vi "SVPWMTimingabcSGL01_src.vi"(0 "A":sgl, 1 "tm":sgl, 2 "tmDIVvdc":sgl, 5 "B":sgl, 7 "C":sgl) -> (4 "U":sgl, 6 "V":sgl, 8 "W":sgl, 14 "Sector":u8)   [LabVIEW 2015]
panel:
  out "tz":sgl
  out "ty":sgl
  out "tx":sgl
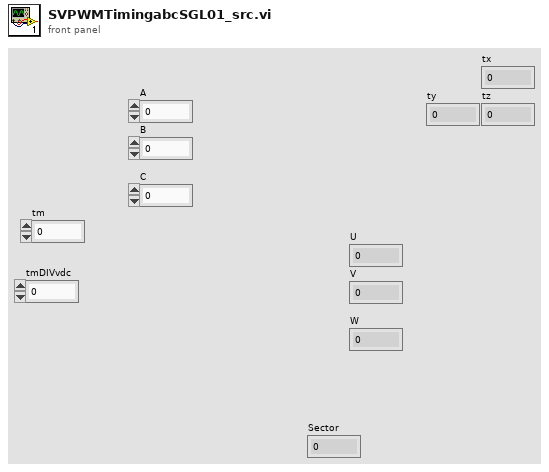
[diagram p1: front panel]
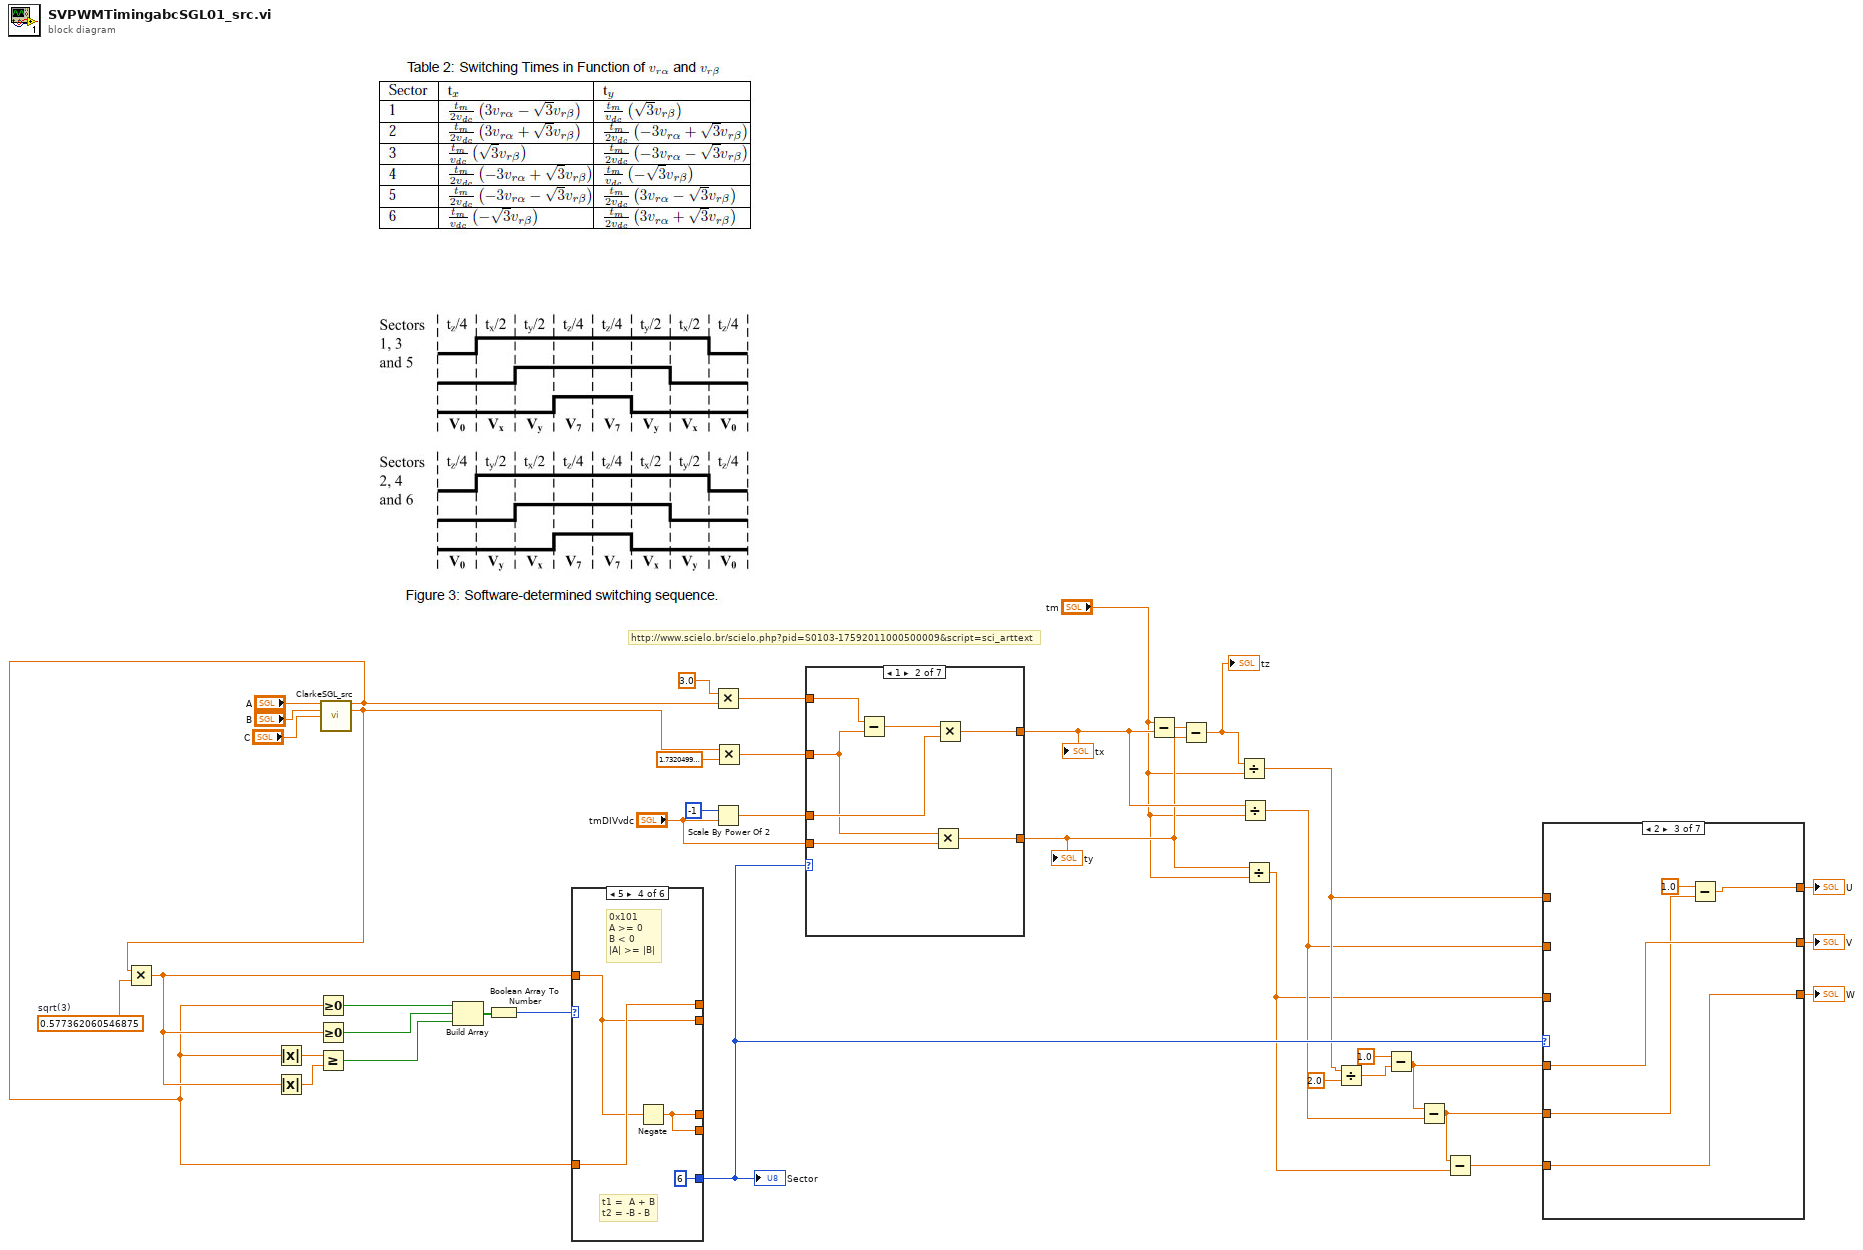
[diagram p0: block diagram]
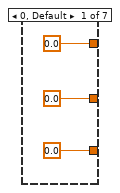
[diagram p2: hidden frame]
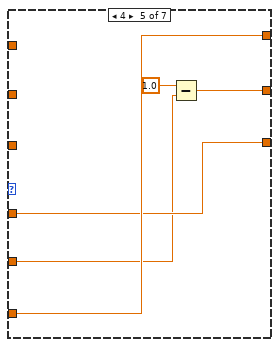
[diagram p5: hidden frame]
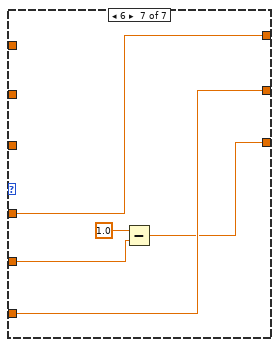
[diagram p7: hidden frame]
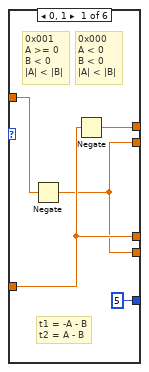
[diagram p8: hidden frame]
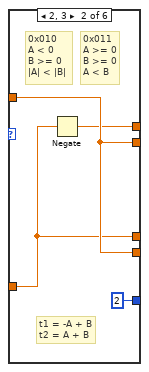
[diagram p9: hidden frame]
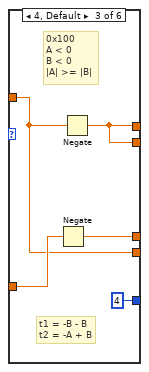
[diagram p10: hidden frame]
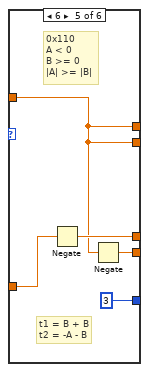
[diagram p11: hidden frame]
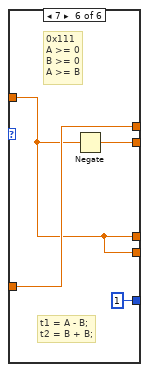
[diagram p12: hidden frame]
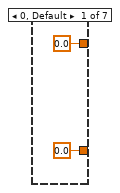
[diagram p13: hidden frame]
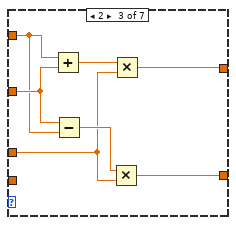
[diagram p14: hidden frame]
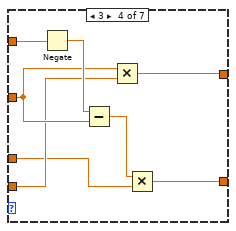
[diagram p15: hidden frame]
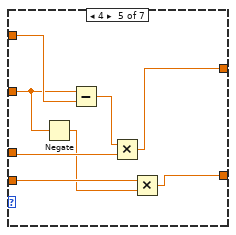
[diagram p16: hidden frame]
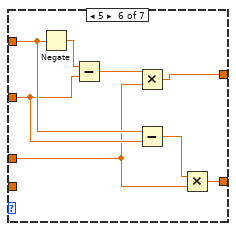
[diagram p17: hidden frame]
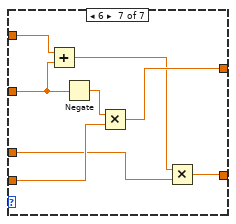
[diagram p18: hidden frame]
diagram:
  w27 = sgl 0.57736206  # sqrt(3)
  # "http://www.scielo.br/scielo.php?pid=S0103-17592011000500009&script=sci_arttext"
  n1 = call "ClarkeSGL_src.vi"("A"="A", "B"="B", "C"="C") -> ("alpha"=w19:sgl, "beta"=w20:sgl)  [unwired: 11 in]
  n2 = Multiply(x=w20, y=w27) -> (x*y=w28:sgl)
  n3 = Absolute Value(x=w19) -> (abs(x)=w26:sgl)
  n4 = Absolute Value(x=w28) -> (abs(x)=w25:sgl)
  n5 = Greater Or Equal To 0?(x=w19) -> (x >= 0?=w23:bool)
  n6 = Greater Or Equal To 0?(x=w28) -> (x >= 0?=w22:bool)
  n7 = Greater Or Equal?(x=w26, y=w25) -> (x >= y?=w21:bool)
  n8 = Build Array(w23, w22, w21) -> (w24:bool[])
  n9 = Boolean Array To Number(Boolean array=w24) -> (number=w29:u8)
  n10 = case shown="5" w29 {
    tunnel: w28 -> [w44 w48 w50 w56 w60 w64]
    tunnel: w19 -> [w42 w46 w53 w57 w62 w65]
    tunnel: [w43 w47 w51 w57 w60 w65] -> _
    tunnel: [w41 w48 w51 w56 w60 w66] -> _
    tunnel: [w42 w46 w52 w55 w61 w64] -> _
    tunnel: [w41 w48 w50 w55 w59 w64] -> _
    tunnel: [u8 5 u8 2 u8 4 u8 6 u8 3 u8 1] -> w17
    frame 0, 1 {
      # "0x000\nA < 0\nB < 0\n|A| < |B|"
      # "t1 = -A - B\nt2 = A - B"
      # "0x001\nA >= 0\nB < 0\n|A| < |B|"
      n11 = Negate(x=w44) -> (-x=w41:sgl)
      n12 = Negate(x=w42) -> (-x=w43:sgl)
    }
    frame 2, 3 {
      # "0x011\nA >= 0\nB >= 0\nA < B"
      # "t1 = -A + B\nt2 = A + B"
      # "0x010\nA < 0\nB >= 0\n|A| < |B|"
      n13 = Negate(x=w46) -> (-x=w47:sgl)
    }
    frame 4, Default {
      # "t1 = -B - B\nt2 = -A + B"
      # "0x100\nA < 0\nB < 0\n|A| >= |B|"
      n14 = Negate(x=w53) -> (-x=w52:sgl)
      n15 = Negate(x=w50) -> (-x=w51:sgl)
    }
    frame 5 {
      # "t1 =  A + B\nt2 = -B - B"
      # "0x101\nA >= 0\nB < 0\n|A| >= |B|"
      n16 = Negate(x=w56) -> (-x=w55:sgl)
    }
    frame 6 {
      # "t1 = B + B\nt2 = -A - B"
      # "0x110\nA < 0\nB >= 0\n|A| >= |B|"
      n17 = Negate(x=w62) -> (-x=w61:sgl)
      n18 = Negate(x=w60) -> (-x=w59:sgl)
    }
    frame 7 {
      # "t1 = A - B;\nt2 = B + B;"
      # "0x111\nA >= 0\nB >= 0\nA >= B"
      n19 = Negate(x=w64) -> (-x=w66:sgl)
    }
  }
  "Sector" <- w17
  n20 = Multiply(x=sgl 3.0, y=w19) -> (x*y=w33:sgl)
  n21 = Scale By Power Of 2(n=i16 -1, x="tmDIVvdc") -> (x*2^n=w31:sgl)
  n22 = Multiply(x=w20, y=sgl 1.73205) -> (x*y=w32:sgl)
  n23 = case shown="1" w17 {
    tunnel: w33 -> [_ w75 w79 w88 w98 w103 w112]
    tunnel: w32 -> [_ w71 w80 w86 w94 w102 w111]
    tunnel: w31 -> [_ w73 w77 w83 w96 w99 w108]
    tunnel: "tmDIVvdc" -> [_ w70 _ w84 w93 _ w109]
    tunnel: [sgl 0.0 w72 w81 w90 w95 w104 w113] -> w15
    tunnel: [sgl 0.0 w69 w76 w89 w91 w101 w107] -> w14
    frame 0, Default {
    }
    frame 1 {
      n24 = Subtract(x=w75, y=w71) -> (x-y=w74:sgl)
      n25 = Multiply(x=w71, y=w70) -> (x*y=w69:sgl)
      n26 = Multiply(x=w74, y=w73) -> (x*y=w72:sgl)
    }
    frame 2 {
      n27 = Add(x=w79, y=w80) -> (x+y=w82:sgl)
      n28 = Subtract(x=w80, y=w79) -> (x-y=w78:sgl)
      n29 = Multiply(x=w78, y=w77) -> (x*y=w76:sgl)
      n30 = Multiply(x=w82, y=w77) -> (x*y=w81:sgl)
    }
    frame 3 {
      n31 = Negate(x=w88) -> (-x=w87:sgl)
      n32 = Subtract(x=w87, y=w86) -> (x-y=w85:sgl)
      n33 = Multiply(x=w86, y=w84) -> (x*y=w90:sgl)
      n34 = Multiply(x=w85, y=w83) -> (x*y=w89:sgl)
    }
    frame 4 {
      n35 = Negate(x=w94) -> (-x=w92:sgl)
      n36 = Subtract(x=w94, y=w98) -> (x-y=w97:sgl)
      n37 = Multiply(x=w97, y=w96) -> (x*y=w95:sgl)
      n38 = Multiply(x=w93, y=w92) -> (x*y=w91:sgl)
    }
    frame 5 {
      n39 = Negate(x=w103) -> (-x=w106:sgl)
      n40 = Subtract(x=w106, y=w102) -> (x-y=w105:sgl)
      n41 = Multiply(x=w105, y=w99) -> (x*y=w104:sgl)
      n42 = Subtract(x=w103, y=w102) -> (x-y=w100:sgl)
      n43 = Multiply(x=w100, y=w99) -> (x*y=w101:sgl)
    }
    frame 6 {
      n44 = Add(x=w112, y=w111) -> (x+y=w110:sgl)
      n45 = Negate(x=w111) -> (-x=w114:sgl)
      n46 = Multiply(x=w114, y=w109) -> (x*y=w113:sgl)
      n47 = Multiply(x=w110, y=w108) -> (x*y=w107:sgl)
    }
  }
  "tx" <- w15
  "ty" <- w14
  n48 = Subtract(x="tm", y=w15) -> (x-y=w18:sgl)
  n49 = Subtract(x=w18, y=w14) -> (x-y=w16:sgl)
  "tz" <- w16
  n50 = Divide(x=w16, y="tm") -> (x/y=w6:sgl)
  n51 = Divide(x=w15, y="tm") -> (x/y=w5:sgl)
  n52 = Divide(x=w14, y="tm") -> (x/y=w4:sgl)
  n53 = Divide(x=w6, y=sgl 2.0) -> (x/y=w9:sgl)
  n54 = Subtract(x=sgl 1.0, y=w9) -> (x-y=w3:sgl)
  n55 = Subtract(x=w3, y=w5) -> (x-y=w2:sgl)
  n56 = Subtract(x=w2, y=w4) -> (x-y=w1:sgl)
  n57 = case shown="2" w17 {
    tunnel: w6 -> [_ _ _ _ _ _ _]
    tunnel: [sgl 0.0 w120 w123 w128 w133 w136 w141] -> w12
    tunnel: w5 -> [_ _ _ _ _ _ _]
    tunnel: [sgl 0.0 w119 w125 w127 w129 w135 w140] -> w11
    tunnel: [sgl 0.0 w118 w124 w126 w132 w134 w137] -> w10
    tunnel: w4 -> [_ _ _ _ _ _ _]
    tunnel: w3 -> [_ w120 w125 w127 w132 w134 w141]
    tunnel: w2 -> [_ w119 w122 w126 w130 w136 w138]
    tunnel: w1 -> [_ w118 w124 w128 w133 w135 w140]
    frame 0, Default {
    }
    frame 1 {
    }
    frame 2 {
      n58 = Subtract(x=sgl 1.0, y=w122) -> (x-y=w123:sgl)
    }
    frame 3 {
    }
    frame 4 {
      n59 = Subtract(x=1.0, y=w130) -> (x-y=w129:dbl)
    }
    frame 5 {
    }
    frame 6 {
      n60 = Subtract(x=1.0, y=w138) -> (x-y=w137:dbl)
    }
  }
  "U" <- w12
  "V" <- w11
  "W" <- w10
